vi "Detect Proximity.vi"(8 "Threshold":dbl, 10 "E current":dbl[](array[numeric]), 11 "E desired":dbl[](array[numeric])) -> (3 "Close Enough?":bool)   [LabVIEW 2018]
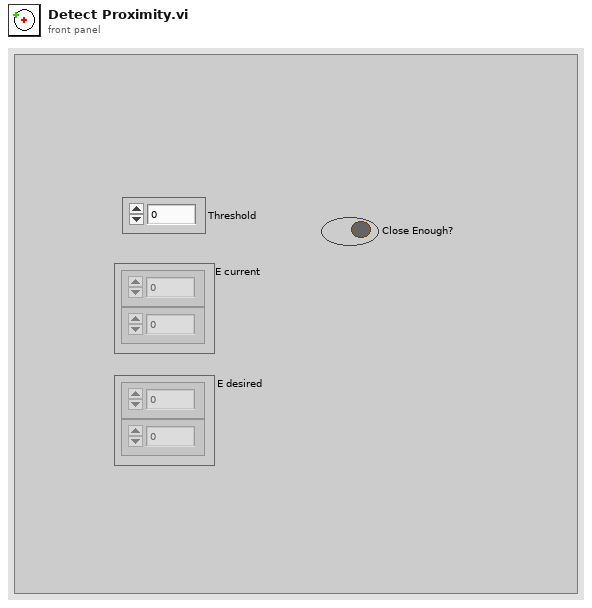
[diagram p1: front panel]
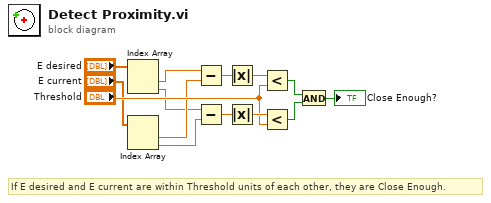
[diagram p0: block diagram]
diagram:
  # "If E desired and E current are within Threshold units of each other, they are Close Enough."
  n1 = Index Array(array="E desired") -> (element #1=w4:dbl, element #2=w2:dbl)  [unwired: 2 in]
  n2 = Index Array(array="E current") -> (element #1=w3:dbl, element #2=w1:dbl)  [unwired: 2 in]
  n3 = Subtract(x=w4, y=w3) -> (x-y=w8:dbl)
  n4 = Subtract(x=w2, y=w1) -> (x-y=w10:dbl)
  n5 = Absolute Value(x=w8) -> (abs(x)=w9:dbl)
  n6 = Absolute Value(x=w10) -> (abs(x)=w11:dbl)
  n7 = Less?(x=w9, y="Threshold") -> (x < y?=w12:bool)
  n8 = Less?(x=w11, y="Threshold") -> (x < y?=w13:bool)
  n9 = And(x=w12, y=w13) -> (x .and. y?=→"Close Enough?":bool)
